vi "TorrosUp.vi"(9 "TorrosCurrPos":bool, 10 "TorrosIn":bool, 11 "ElevBasePosIn":T1) -> (2 "TorrosOut":bool, 3 "ElevBasePosOut":T1)   [LabVIEW 2018]
uses:
  ElevBasePos.ctl
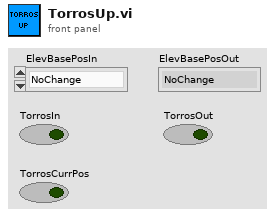
[diagram p1: front panel]
types:
  T1 = typedef "ElevBasePos.ctl" = enum16{"NoChange", "ShipHatch", "RocketHatch", "Carry", "Cargo"}
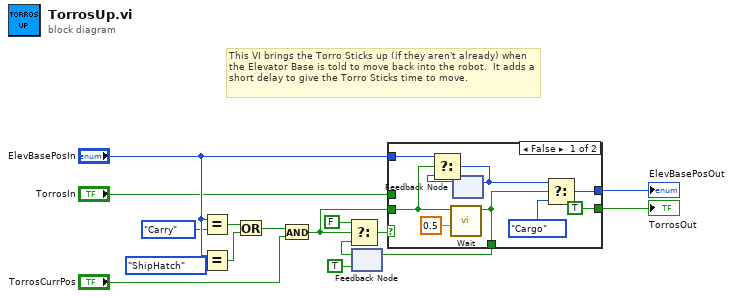
[diagram p0: block diagram]
diagram:
  # "This VI brings the Torro Sticks up (if they aren't already) when the Elevator Base is told to move back into the robot.  It adds a short delay to give the Torro Sticks time to move."
  n1 = Equal?(x="ElevBasePosIn", y=ElevBasePos."Carry") -> (x = y?=w11:bool)
  n2 = Equal?(x="ElevBasePosIn", y=ElevBasePos."ShipHatch") -> (x = y?=w12:bool)
  n3 = Or(x=w11, y=w12) -> (x .or. y?=w13:bool)
  n4 = And(x=w13, y="TorrosCurrPos") -> (x .and. y?=w14:bool)
  n5 = feedback #1(TRUE ("Completed")) -> (w8:bool)
  n6 = Select(t=FALSE, s=w14, f=w8) -> (s? t:f=w10:bool)
  n7 = case shown="False" w10 {
    selector: w10 -> [_ w26]
    tunnel: "TorrosIn" -> [_ w27]
    tunnel: [TRUE w27] -> w6
    tunnel: [w20 w26] -> w9
    tunnel: w14 -> [w21 _]
    tunnel: "ElevBasePosIn" -> [w22 w28]
    tunnel: [w17 w28] -> w16
    frame False {
      n8 = call "Wait.vi"("Target Time (s)"=0.5, "Start Timer?"=w21) -> ("Completed"=w20:bool)  [unwired: 8 in, 1 out]
      n9 = feedback #2() -> (w23:T1)  [unwired: 1 in]
      n10 = Select(t=w22, s=w21, f=w23) -> (s? t:f=w19:T1)
      n11 = feedback-in #2(w19) -> ()
      n12 = Select(t=w19, s=w20, f=ElevBasePos."Cargo") -> (s? t:f=w17:T1)
    }
    frame True {
    }
  }
  "ElevBasePosOut" <- w16
  "TorrosOut" <- w6
  n13 = feedback-in #1(w9) -> ()
